vi "Generate Unique Header.vi"(8 "error in (no error)":errorcluster, 11 "CRDS Cell Data in":refnum<class "CRDS Cell Data.lvclass">) -> (0 "error out":errorcluster, 2 "Header":string[](array[string]), 3 "CRDS Cell Data out":refnum<class "CRDS Cell Data.lvclass">)   [LabVIEW 2014, in "CRDS Lib.lvlib" / "CRDS Cell Data.lvclass"]
uses:
  CRDS Cell Data.lvclass
  Data/Data.lvclass/Data.ctl
  Data/Read Data ID.vi
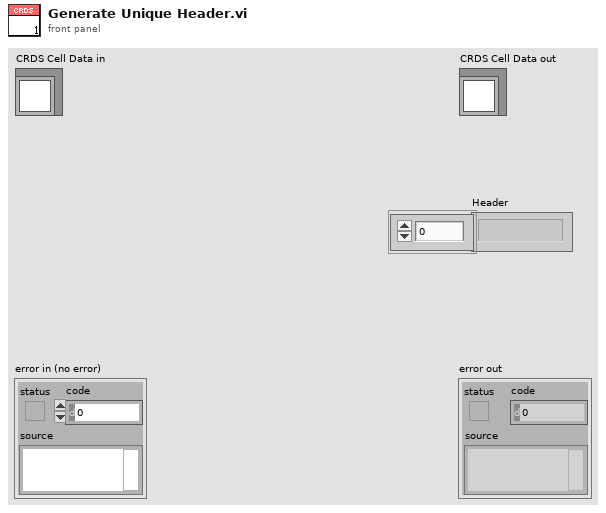
[diagram p1: front panel]
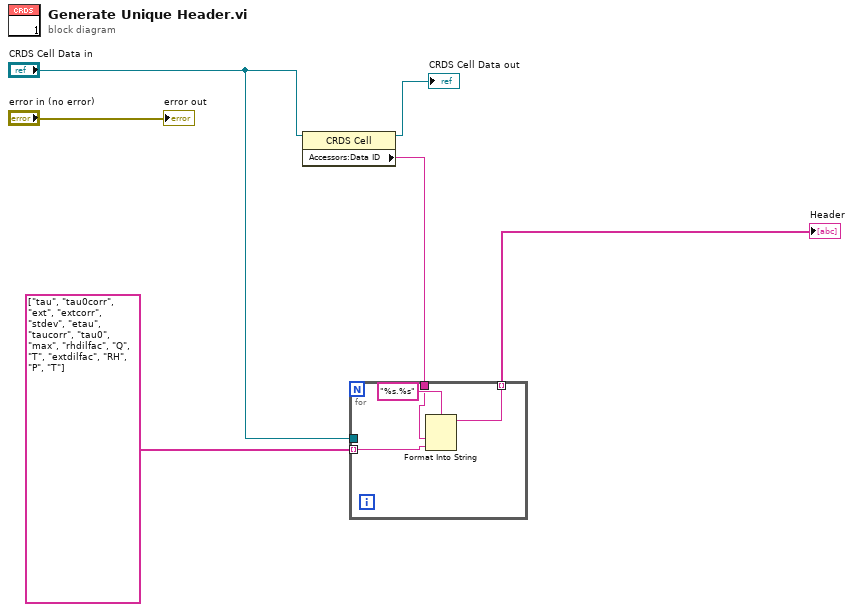
[diagram p0: block diagram]
diagram:
  n1 = property class="CRDS Cell"(reference="CRDS Cell Data in") -> (reference out=→"CRDS Cell Data out":refnum<class "CRDS Cell Data.lvclass">, "Accessors:Data ID"=w2:string)  [unwired: 1 in, 1 out]
  n2 = for {
    tunnel: "CRDS Cell Data in" -> [_]
    tunnel: string[] ["tau", "tau0corr", "ext", "extcorr", "stdev", "etau", "taucorr", "tau0", "max", "rhdilfac", "Q", "T", "extdilfac", "RH", "P", "T"] -> [w10] mode=indexing
    tunnel: [w8] -> w4 mode=indexing
    tunnel: w2 -> [w7]
    n3 = Format Into String(format string="%s.%s", w7, w10) -> (resulting string=w8:string)  [unwired: 2 in, 1 out]
  }
  "Header" <- w4
  "error out" <- "error in (no error)"
